vi "CarMoveUp.vi"(8 "Y+X":i32=180, 9 "Y":i32=80, 10 "speed":u32=1 min=1, 11 "Boolean in":refnum<vi>) -> ()   [LabVIEW 2023]
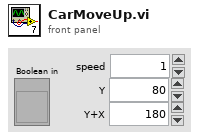
[diagram p1: front panel]
types:
  T1 = typedef "LVPositionTypeDef.ctl" = cluster{"Left":i32, "Top":i32}
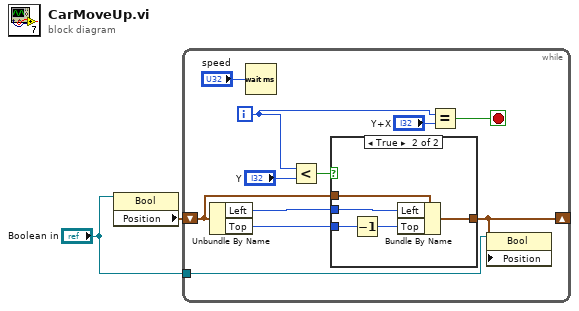
[diagram p0: block diagram]
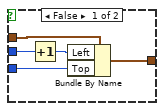
[diagram p2: hidden frame]
diagram:
  n1 = property on="Property Node" class="Bool"(reference="Boolean in") -> ("Position"=w2:T1)  [unwired: 1 in, 2 out]
  n2 = while {
    shift-right: [w10] -> _
    shift-left: w2 -> [w13]
    tunnel: "Boolean in" -> [w5]
    i -> [w3]
    stop <- w11 stop-if-true
    n3 = Unbundle By Name(w13) -> ("Left"=w9:i32, "Top"=w8:i32)
    n4 = Wait (ms)(milliseconds to wait="speed") -> ()  [unwired: 1 out]
    n5 = Less?(x=w3, y="Y") -> (x < y?=w6:bool)
    n6 = case shown="True" w6 {
      tunnel: w13 -> [w18 w20]
      tunnel: [w17 w21] -> w10
      tunnel: w9 -> [w16 w22]
      tunnel: w8 -> [w15 w23]
      frame False {
        n7 = Increment(x=w16) -> (x+1=w14:i32)
        n8 = Bundle By Name(cluster=w18, "Left"=w14, "Top"=w15) -> (w17:T1)
      }
      frame True {
        n9 = Decrement(x=w23) -> (x-1=w19:i32)
        n10 = Bundle By Name(cluster=w20, "Left"=w22, "Top"=w19) -> (w21:T1)
      }
    }
    n11 = Equal?(x=w3, y="Y+X") -> (x = y?=w11:bool)
    n12 = property on="Property Node" class="Bool"(reference=w5, "Position"=w10) -> ()  [unwired: 1 in, 2 out]
  }
